vi "Meas_Sweep.vi"(0 "SPU":refnum<k24>, 1 "Flag_215":bool, 2 "MPM":refnum<k24>[](array[refnum]), 3 "Data_struct":refnum<k24>[](array[refnum]), 4 "TSL":refnum<k24>, 5 "错误输入（无错误）":errorcluster, 7 "ILSTS":refnum<k24>, 8 "Flag_213":bool, 11 "Meas_monitor_struct":refnum<k24>[](array[refnum]), 12 "Meas_rang":i32[](array[numeric])) -> (19 "错误输出":errorcluster)   [LabVIEW 2017]
uses:
  D:/test/ILSTS/LV_IL/LV_IL_Sample_x64/DLL/InstrumentDLL.dll
  DLL/InstrumentDLL.dll
  D:/test/ILSTS/LV_IL/LV_IL_Sample_x64/DLL/STSProcess.dll
  DLL/STSProcess.dll
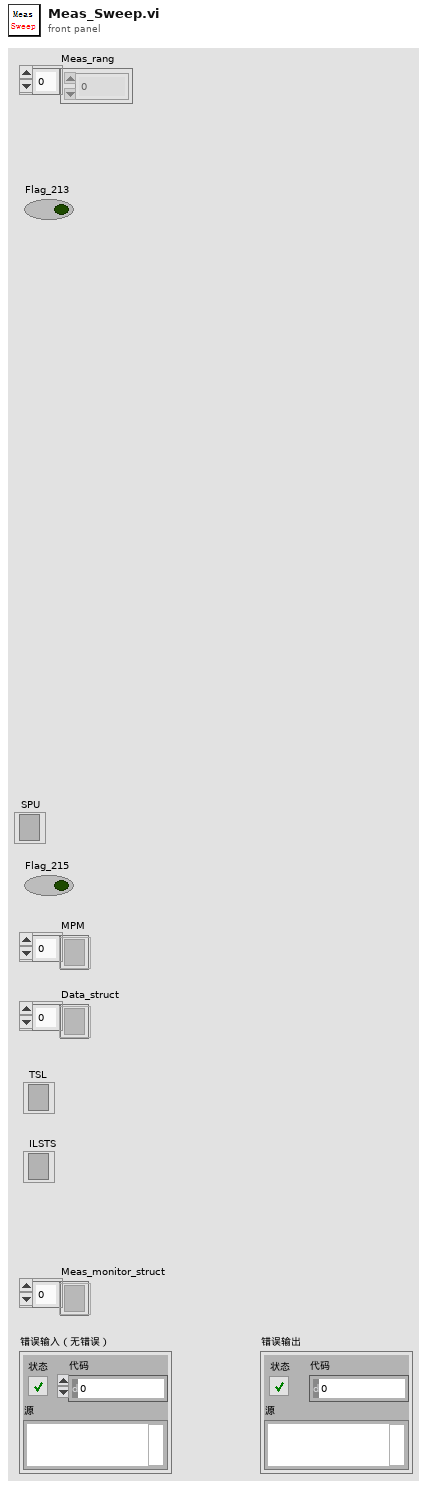
[diagram p1: front panel]
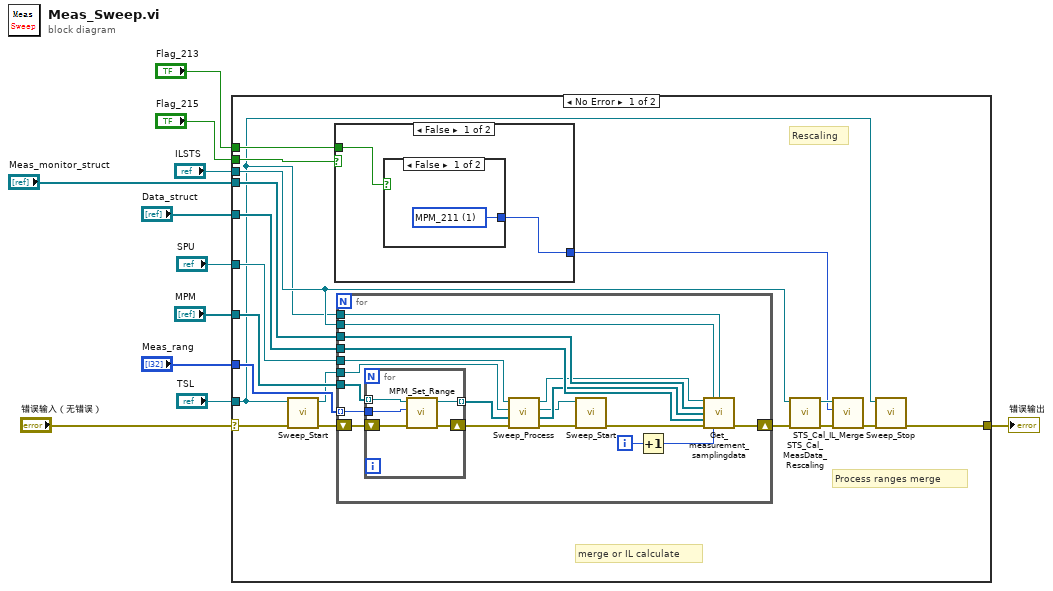
[diagram p0: block diagram]
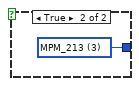
[diagram p2: hidden frame]
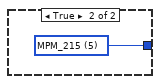
[diagram p3: hidden frame]
diagram:
  n1 = case shown="No Error" "错误输入（无错误）" {
    selector: "错误输入（无错误）" -> [w20 w59]
    tunnel: [w29 w59] -> w11
    tunnel: "Flag_213" -> [w28 _]
    tunnel: "Flag_215" -> [w27 _]
    tunnel: "MPM" -> [w26 _]
    tunnel: "Data_struct" -> [w25 _]
    tunnel: "Meas_monitor_struct" -> [w24 _]
    tunnel: "SPU" -> [w23 _]
    tunnel: "ILSTS" -> [w22 _]
    tunnel: "Meas_rang" -> [w21 _]
    tunnel: "TSL" -> [w12 _]
    frame No Error {
      # "Rescaling"
      # "Process ranges merge"
      # "merge or IL calculate"
      n2 = call "Sweep_Start.vi"("error in (no error)"=w20, ".NET Reference in"=w12) -> ("error out"=w19:errorcluster, "Reference out"=w18:refnum<k24>)  [unwired: 8 in]
      n3 = case shown="False" w27 {
        tunnel: [w31 w34] -> w14
        tunnel: w28 -> [w30 _]
        frame False {
          n4 = case shown="False" w30 {
            tunnel: [w32 w33] -> w31
            frame False {
              w32 = 1 items=["MPM_10"=0, "MPM_211"=1, "MPM_212"=2, "MPM_213"=3, "MPM_215"=5] ("type")
            }
            frame True {
              w33 = 3 items=["MPM_10"=0, "MPM_211"=1, "MPM_212"=2, "MPM_213"=3, "MPM_215"=5] ("type")
            }
          }
        }
        frame True {
          w34 = 5 items=["MPM_10"=0, "MPM_211"=1, "MPM_212"=2, "MPM_213"=3, "MPM_215"=5] ("type")
        }
      }
      n5 = for {
        tunnel: w21 -> [w52] mode=indexing
        tunnel: w26 -> [w44]
        tunnel: w18 -> [w49]
        tunnel: w23 -> [w45]
        tunnel: w22 -> [w48]
        tunnel: w24 -> [w47]
        tunnel: w25 -> [w46]
        shift-right: [w43] -> w13
        shift-left: w19 -> [w53]
        tunnel: w12 -> [w35]
        i -> [w42]
        n6 = for {
          tunnel: w44 -> [w58] mode=indexing
          tunnel: w52 -> [w55]
          shift-right: [w56] -> w51
          shift-left: w53 -> [w57]
          tunnel: [w54] -> w41 mode=indexing
          n7 = call "MPM_Set_Range.vi"("error in (no error)"=w57, "Range All"=w55, ".NET Reference in"=w58) -> ("error out"=w56:errorcluster, "Reference out"=w54:refnum<k24>)  [unwired: 7 in]
        }
        n8 = call "Sweep_Process.vi"("错误输入（无错误）"=w51, "MPM"=w41, "TSL"=w49, "SPU"=w45) -> ("error out"=w50:errorcluster, "MPM out"=w40:refnum<k24>[], "TSL out"=w39:refnum<k24>, "SPU out"=w38:refnum<k24>)  [unwired: 4 in]
        n9 = call "Sweep_Start.vi"("error in (no error)"=w50, ".NET Reference in"=w39) -> ("error out"=w37:errorcluster)  [unwired: 8 in, 1 out]
        n10 = Increment(x=w42) -> (x+1=w36:i32)
        n11 = call "Get_measurement_samplingdata.vi"("SPU"=w38, "STSProcess.ILSTS"=w48, "TSL"=w35, "Meas_monitor_struct"=w47, "MPM"=w40, "Data_struct"=w46, "错误输入（无错误）"=w37, "SweepCount"=w36) -> ("error out"=w43:errorcluster)  [unwired: 7 in]
      }
      n12 = call "STS_Cal_MeasData_Rescaling.vi"("错误输入（无错误）"=w13, ".NET引用句柄输入"=w22) -> ("error out"=w15:errorcluster, "引用输出"=w16:refnum<k24>)  [unwired: 8 in]
      n13 = call "STS_Cal_IL_Merge.vi"("错误输入（无错误）"=w15, "type"=w14, ".NET引用句柄输入"=w16) -> ("error out"=w17:errorcluster)  [unwired: 7 in, 1 out]
      n14 = call "Sweep_Stop.vi"("error in (no error)"=w17, ".NET Reference in"=w12) -> ("error out"=w29:errorcluster)  [unwired: 8 in, 1 out]
    }
    frame Error {
    }
  }
  "错误输出" <- w11
